vi "Test Valid Registration.vi"() -> ()   [LabVIEW 2024]
uses:
  Sift API/Sift Client.lvclass
  Sift API/Types/Data Type.ctl
  Sift Client.lvlib
  Mock Sift Proxy Server/Mock Sift Proxy Server.lvclass
panel:
  out "Server Error":errorcluster
  out "Success":bool
  out "Error 2":errorcluster
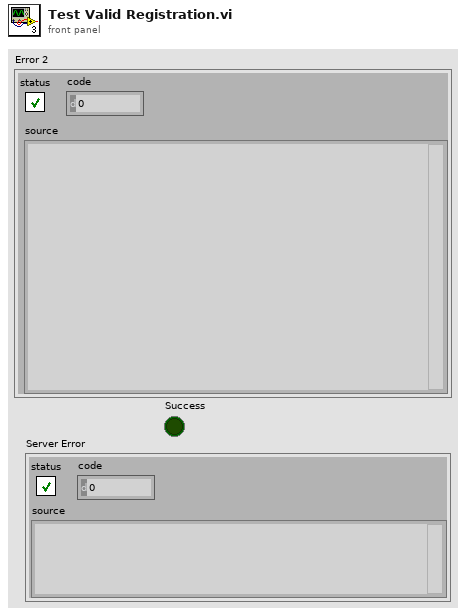
[diagram p1: front panel]
types:
  T1 = typedef "Sift Client.lvlib/Data Type.ctl" = enum8{"double", "float", "uint64", "int64", "uint32", "int32", "bool", "bit field", "enum", "string"}
  T2 = typedef "Sift Client.lvlib/JSON Response.ctl" = cluster{"status":bool, "data":variant}
  T3 = typedef "Sift Client.lvlib/Channel Config.ctl" = cluster{"name":string, "data_type":T1, "description":string, "component":string, "unit":string, "bit_field_elements":T4[], "enum_types":T5[]}
  T4 = typedef "Sift Client.lvlib/Bit Field.ctl" = cluster{"index":u32, "bit_count":u32, "name":string}
  T5 = typedef "Sift Client.lvlib/Enum.ctl" = cluster{"Key":u32, "Name":string}
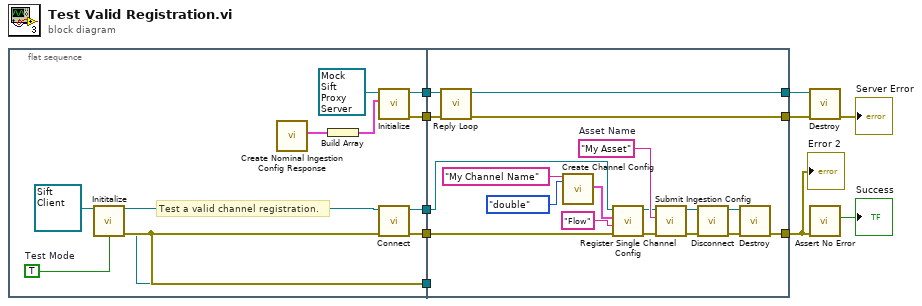
[diagram p0: block diagram]
diagram:
  n1 = flat-sequence {
    tunnel: [w21] -> w11
    tunnel: [w18] -> w10
    tunnel: [w17] -> w9
    tunnel: [w16] -> w8
    tunnel: [w15] -> w7
    tunnel: [w14] -> w6
    tunnel: [w29] -> w4
    tunnel: w11 -> [w30]
    tunnel: [w38] -> w3
    tunnel: w10 -> [_]
    tunnel: w9 -> [_]
    tunnel: w8 -> [w28]
    tunnel: w7 -> [w27]
    tunnel: w6 -> [w24]
    tunnel: [w23] -> w2
    frame #0 {
      w19 = TRUE  # Test Mode
      # "Test a valid channel registration."
      n2 = call-dynamic "Inititalize.vi"("Sift Client in"=refnum<class "Sift Client.lvclass"> refnum ("Sift Client.lvlib:Sift Client.lvclass"), "Test Mode"=w19) -> ("Sift Client out"=w17:refnum<class "Sift Client.lvclass">, "error out"=w18:errorcluster)  [unwired: 12 in]
      n3 = call "Create Nominal Ingestion Config Response.vi"() -> ("output cluster"=w13:T2)  [unwired: 11 in]
      n4 = Build Array(w13) -> (w12:T2[])
      n5 = call-dynamic "Initialize.vi"("Mock Replies"=w12, "Mock Sift Proxy Server in"=refnum<class "Mock Sift Proxy Server.lvclass"> refnum ("Mock Sift Proxy Server.lvclass")) -> ("error out"=w14:errorcluster, "Mock Sift Proxy Server out"=w21:refnum<class "Mock Sift Proxy Server.lvclass">)  [unwired: 8 in]
      n6 = call-dynamic "Connect.vi"("error in (no error)"=w18, "Sift Client in"=w17) -> ("error out"=w16:errorcluster, "Sift Client out"=w15:refnum<class "Sift Client.lvclass">)  [unwired: 7 in, 1 out]
    }
    frame #1 {
      w34 = "My Asset"  # Asset Name
      n7 = call-dynamic "Reply Loop.vi"("error in (no error)"=w24, "Mock Sift Proxy Server in"=w30) -> ("error out"=w23:errorcluster, "Mock Sift Proxy Server out"=w29:refnum<class "Mock Sift Proxy Server.lvclass">)  [unwired: 8 in]
      n8 = call "Create Channel Config.vi"("Name"="My Channel Name", "Data Type"=Data_Type."double" ("Enum")) -> ("Output"=w35:T3)  [unwired: 17 in]
      n9 = call-dynamic "Register Single Channel Config.vi"("error in (no error)"=w28, "Flow Name"="Flow", "Channel Config"=w35, "Sift Client in"=w27) -> ("error out"=w39:errorcluster, "Sift Client out"=w32:refnum<class "Sift Client.lvclass">)  [unwired: 6 in]
      n10 = call-dynamic "Submit Ingestion Config.vi"("error in (no error)"=w39, "Asset Name"=w34, "Sift Client in"=w32) -> ("error out"=w40:errorcluster, "Sift Client out"=w31:refnum<class "Sift Client.lvclass">)  [unwired: 6 in, 1 out]
      n11 = call-dynamic "Disconnect.vi"("error in (no error)"=w40, "Sift Client in"=w31) -> ("error out"=w25:errorcluster, "Sift Client out"=w26:refnum<class "Sift Client.lvclass">)  [unwired: 8 in]
      n12 = call-dynamic "Destroy.vi"("error in (no error)"=w25, "Sift Client in"=w26) -> ("error out"=w38:errorcluster)  [unwired: 8 in, 1 out]
    }
  }
  n13 = call-dynamic "Destroy.vi"("error in (no error)"=w2, "Mock Sift Proxy Server in"=w4) -> ("error out"=→"Server Error":errorcluster)  [unwired: 8 in, 1 out]
  n14 = call "Assert No Error.vi"("Error"=w3) -> ("Success"=→"Success":bool)  [unwired: 10 in]
  "Error 2" <- w3
